vi "Get All Projects.vi"(8 "error in (no error)":errorcluster, 11 "Projects in":refnum<class "Projects.lvclass">) -> (0 "error out":errorcluster, 2 "Projects":string[](array[string]), 3 "Projects out":refnum<class "Projects.lvclass">)   [LabVIEW 2020, in "Projects.lvclass"]
doc: "Reads out the projects from the Map. If no projects are present then the Projects output will be an empty array.\n\n03/2025 Erich Schlieper"
uses:
  Projects.lvclass
  Projects.lvclass/Projects.ctl
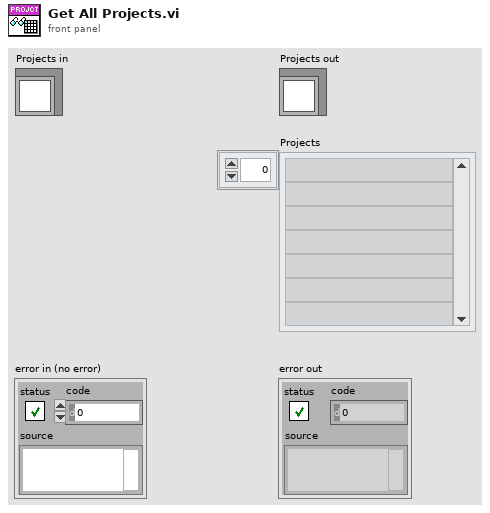
[diagram p1: front panel]
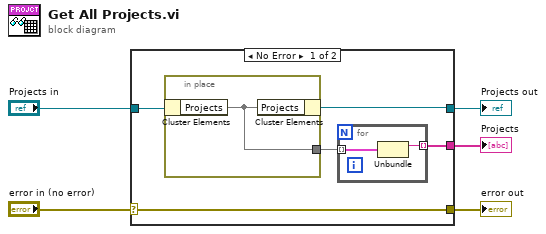
[diagram p0: block diagram]
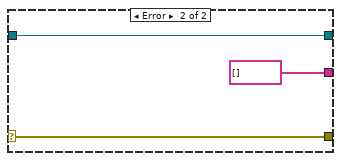
[diagram p2: hidden frame]
diagram:
  n1 = case shown="No Error" "error in (no error)" {
    selector: "error in (no error)" -> [w9 w16]
    tunnel: [w9 w16] -> w4
    tunnel: [w8 w15] -> w2
    tunnel: "Projects in" -> [w10 w15]
    tunnel: [w6 string[] []] -> w1
    frame No Error {
      n2 = in-place {
        in-place-border: [w13] -> w7
        n3 = in-place-cluster #1(w10) -> ("Projects"=w13:map{string, set{string}})
        n4 = in-place-cluster #1("Projects"=w13) -> (w8:refnum<class "Projects.lvclass">)
      }
      n5 = for {
        tunnel: [w11] -> w6 mode=indexing
        tunnel: w7 -> [w12] mode=indexing
        n6 = Unbundle(w12) -> (w11:string)  [unwired: 1 out]
      }
    }
    frame Error {
    }
  }
  "error out" <- w4
  "Projects out" <- w2
  "Projects" <- w1
